vi "DAC go.vi"(4 "ntimes":u32=250001, 5 "time step":dbl=1.0, 7 "Input Array":waveform(dbl)[](array[waveform])=[{"t0"=timestamp(0 s since 1904-01-01), "dt"=1e-05, "Y"=array[250002 elements]}, {"t0"=timestamp(0 s since 1904-01-01), "dt"=1e-05, "Y"=array[250002 elements]}, {"t0"=timestamp(0 s since 1904-01-01), "dt"=1e-05, "Y"=array[250002 elements]}, {"t0"=timestamp(0 s since 1904-01-01), "dt"=1e-05, "Y"=array[250002 elements]}, {"t0"=timestamp(0 s since 1904-01-01), "dt"=1e-05, "Y"=array[250002 elements]}, {"t0"=timestamp(0 s since 1904-01-01), "dt"=1e-05, "Y"=array[250002 elements]}, {"t0"=timestamp(0 s since 1904-01-01), "dt"=1e-05, "Y"=array[250002 elements]}, {"t0"=timestamp(0 s since 1904-01-01), "dt"=1e-05, "Y"=array[250002 elements]}]) -> (0 "error out":errorcluster, 3 "task out":refnum<k21>)   [LabVIEW 2017]
doc: "This subVI makes the DAC go, including configuring the trigger and writing the data to the board. It does not wait for execution."
uses:
  <vilib>/DAQmx/write.llb/DAQmx Write (Analog 1D Wfm NChan NSamp).vi
  globals/RIO and DAC defaults global.vi
  <vilib>/DAQmx/create/channels.llb/DAQmx Create Channel (AO-Voltage-Basic).vi
  <vilib>/DAQmx/configure/timing.llb/DAQmx Timing (Sample Clock).vi
  <vilib>/DAQmx/miscellaneous.llb/DAQmx Fill In Error Info.vi
  <vilib>/DAQmx/configure/trigger.llb/DAQmx Start Trigger (Digital Edge).vi
panel:
  out "number of samples written per channel":u32
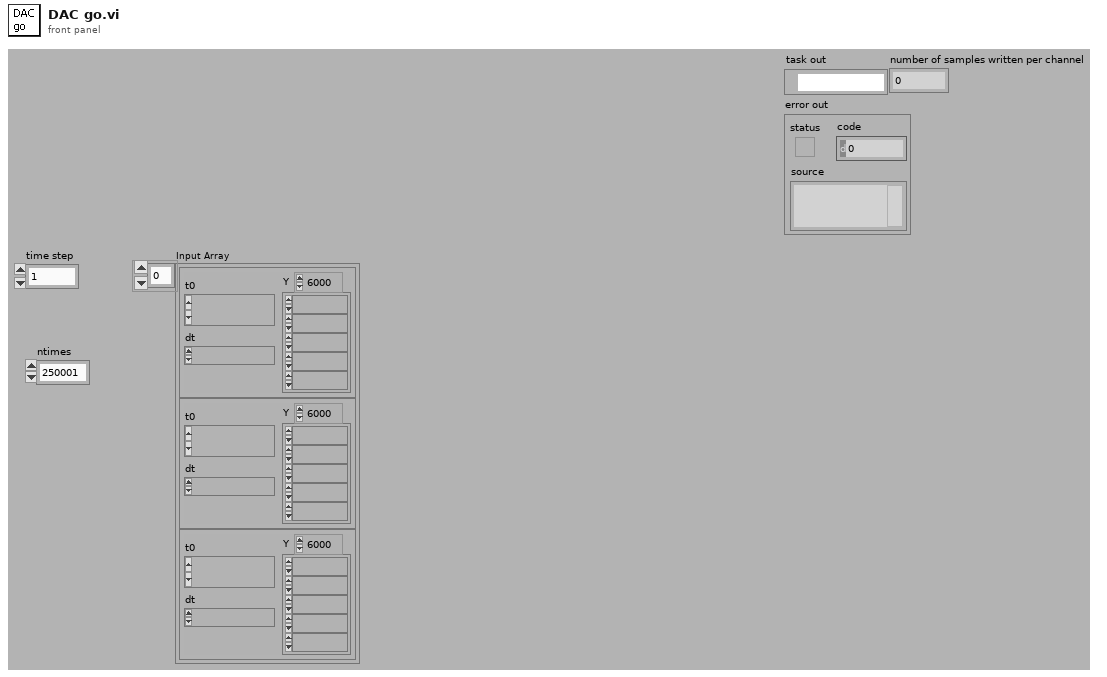
[diagram p1: front panel]
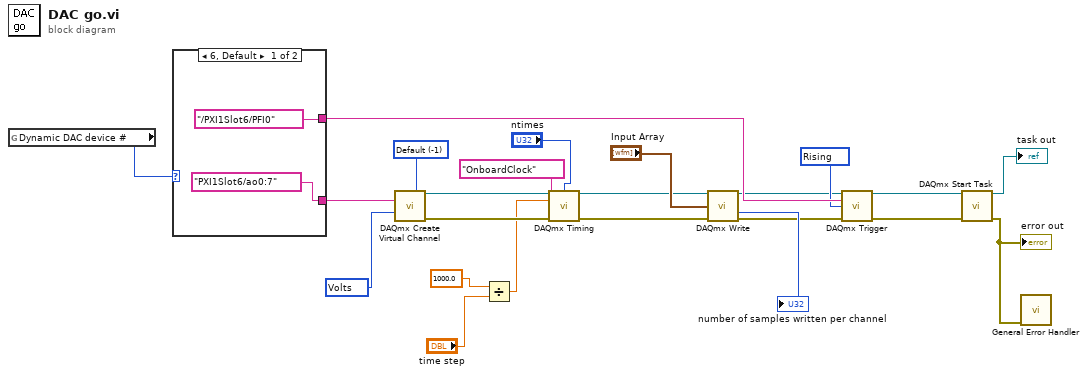
[diagram p0: block diagram]
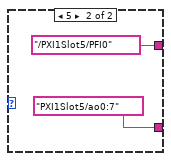
[diagram p2: hidden frame]
diagram:
  w17 = 10348 items=["Volts"=10348, "From Custom Scale"=10065] ("units")
  w18 = -1 items=["Default"=-1, "RSE"=10083, "Differential"=10106, "Pseudodifferential"=12529] ("output terminal configuration")
  w20 = 10280 items=["Rising"=10280, "Falling"=10171] ("edge")
  n1 = global read "RIO and DAC defaults global.vi" "Dynamic DAC device #"() -> (w23:i16)
  n2 = case shown="6, Default" w23 {
    tunnel: [tag "PXI1Slot6/ao0:7" ("physical channels") tag "PXI1Slot5/ao0:7" ("physical channels")] -> w22
    tunnel: [tag "/PXI1Slot6/PFI0" ("source") tag "/PXI1Slot5/PFI0" ("source")] -> w21
    frame 6, Default {
    }
    frame 5 {
    }
  }
  n3 = call-poly <vilib>:"DAQmx Create Virtual Channel.vi"("output terminal configuration"=w18, "physical channels"=w22, "units"=w17) -> ("task out"=w16:refnum<k21>, "error out"=w14:errorcluster)  [unwired: 11 in]
  n4 = Divide(x=1000.0 ("y"), y="time step") -> (x/y=w13:dbl)
  n5 = call-poly <vilib>:"DAQmx Timing.vi"("task/channels in"=w16, "samples per channel"="ntimes", "rate"=w13, "source"=tag "OnboardClock", "error in"=w14) -> ("task out"=w7:refnum<k21>, "error out"=w6:errorcluster)  [unwired: 9 in]
  n6 = call-poly <vilib>:"DAQmx Write.vi"("task/channels in"=w7, "data"="Input Array", "error in"=w6) -> ("task out"=w5:refnum<k21>, "number of samples written per channel"=→"number of samples written per channel":u32, "error out"=w4:errorcluster)  [unwired: 10 in]
  n7 = call-poly <vilib>:"DAQmx Trigger.vi"("task/channels in"=w5, "source"=w21, "edge"=w20, "error in"=w4) -> ("task out"=w3:refnum<k21>, "error out"=w2:errorcluster)  [unwired: 10 in]
  n8 = call <vilib>:"DAQmx Start Task.vi"("task/channels in"=w3, "error in"=w2) -> ("task out"=→"task out":refnum<k21>, "error out"=w8:errorcluster)  [unwired: 12 in]
  "error out" <- w8
  n9 = call <vilib>:"General Error Handler.vi"("error in (no error)"=w8) -> ()  [unwired: 10 in, 5 out]
